vi "OpenScan-packed DRAM-FPGA.vi"() -> ()   [LabVIEW 2015]
uses:
  <vilib>/eio/EIONode/EIONode.xnode
  <vilib>/rvi/eio/common/nirviEmuTemplateMethod_errors.vi
  OpenScan Labview code_20170126/Global_Sample per Frame.vi
  Grobal Variable_Pixel Clock.vi
panel:
  out "Imaging data unpacked for Kalman":u32
  out "Max DRAM address _indicator":u32
  out "Imaging data averaged":u32
  out "Imaging data DRAM address":u32
  in  "Max DRAM address":u32
  in  "Frame number":i32
  out "Number of frames indicator":i32
  out "Waveform output loop count_indicator":i32
  out "Num of elements_indicator":u32=512000
  out "Waiting?":bool=TRUE
  out "Stopping?":bool=TRUE
  out "Frame address_Global":u32
  out "FPGA stop":bool
  out "FPGA loop count":i32
  out "Frams done_indicator":i32
  out "Num of data":u32
  out "Kalman Imaging data address":u32
  out "Display imaging data address":u32
  out "Galvo signal readed_indicator":u32
  in  "Number of frames":i32
  out "Samples acquired":u32
  out "Samples per frame_Global":u32
  out "Frame waveform output finish?":bool
  out "Frame acquisition finish?":bool
  out "image data address indicator":u32
  out "Data indicator":u32
  out "Address counter":u32
  out "Pixel clock_indicator":bool
  out "Frame address_indicator":u32
  out "Averaged image displayed? _indicator":bool
  out "Scanning?":bool
  out "loop count":i32
  out "Display_frames done":i32
  out "Averaged data address":u32
  out "Frame imaging data averaged?":bool
  out "Averaged image displayed?":bool
  in  "Kalman gain":fxp<+,16,1>=0.1015625
  in  "Filter gain":fxp<+,16,0>=0.8000030517578125
  in  "Ready to Scan":bool
  out "Pixel clock (Indicator)":bool
  out "Image averaging done?":bool
  in  "Samples per frame control":u32=262144
  out "Data":u32
  out "Galvo signal readed":u32
  out "Request address":u32
  out "Line clock":bool
  in  "Pixel clock_pulse width(tick)":i32
  in  "Resolution":i32
  in  "Pixel pulse_initial delay":i32
  in  "Frame retrace time":u32 caption="Frame retrace time (ms)"
  in  "Num of undershoot":i32
  in  "Elements per line":i32
  in  "Num of elements":u32
  in  "Pixel time (tick)":i32
  out "Write DRAM done?":bool
  in  "Total elements":u32
  out "Frame Galvo signal write done?":bool
  in  "max addr":u32=1024
  in  "Write DRAM enable?":bool
  in  "Write Frame Galvo signal?":bool
  # "Waveform Data Loading"
  # "Photon Counting"
  # "Waveform Generation"
  # "Controller"
  # "Indicator"
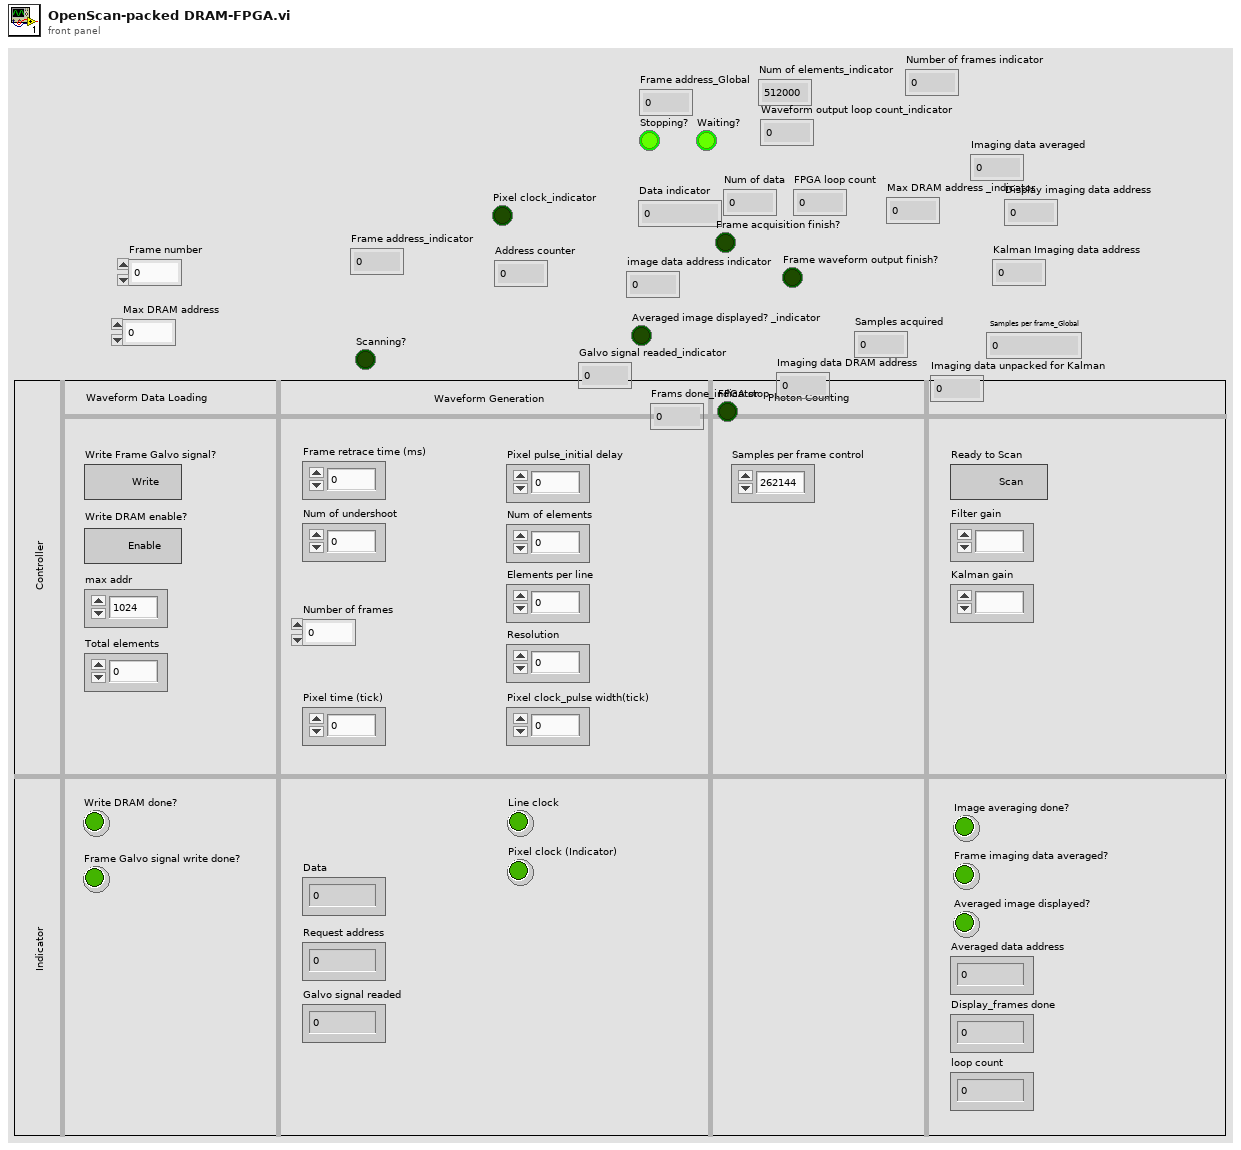
[diagram p1: front panel]
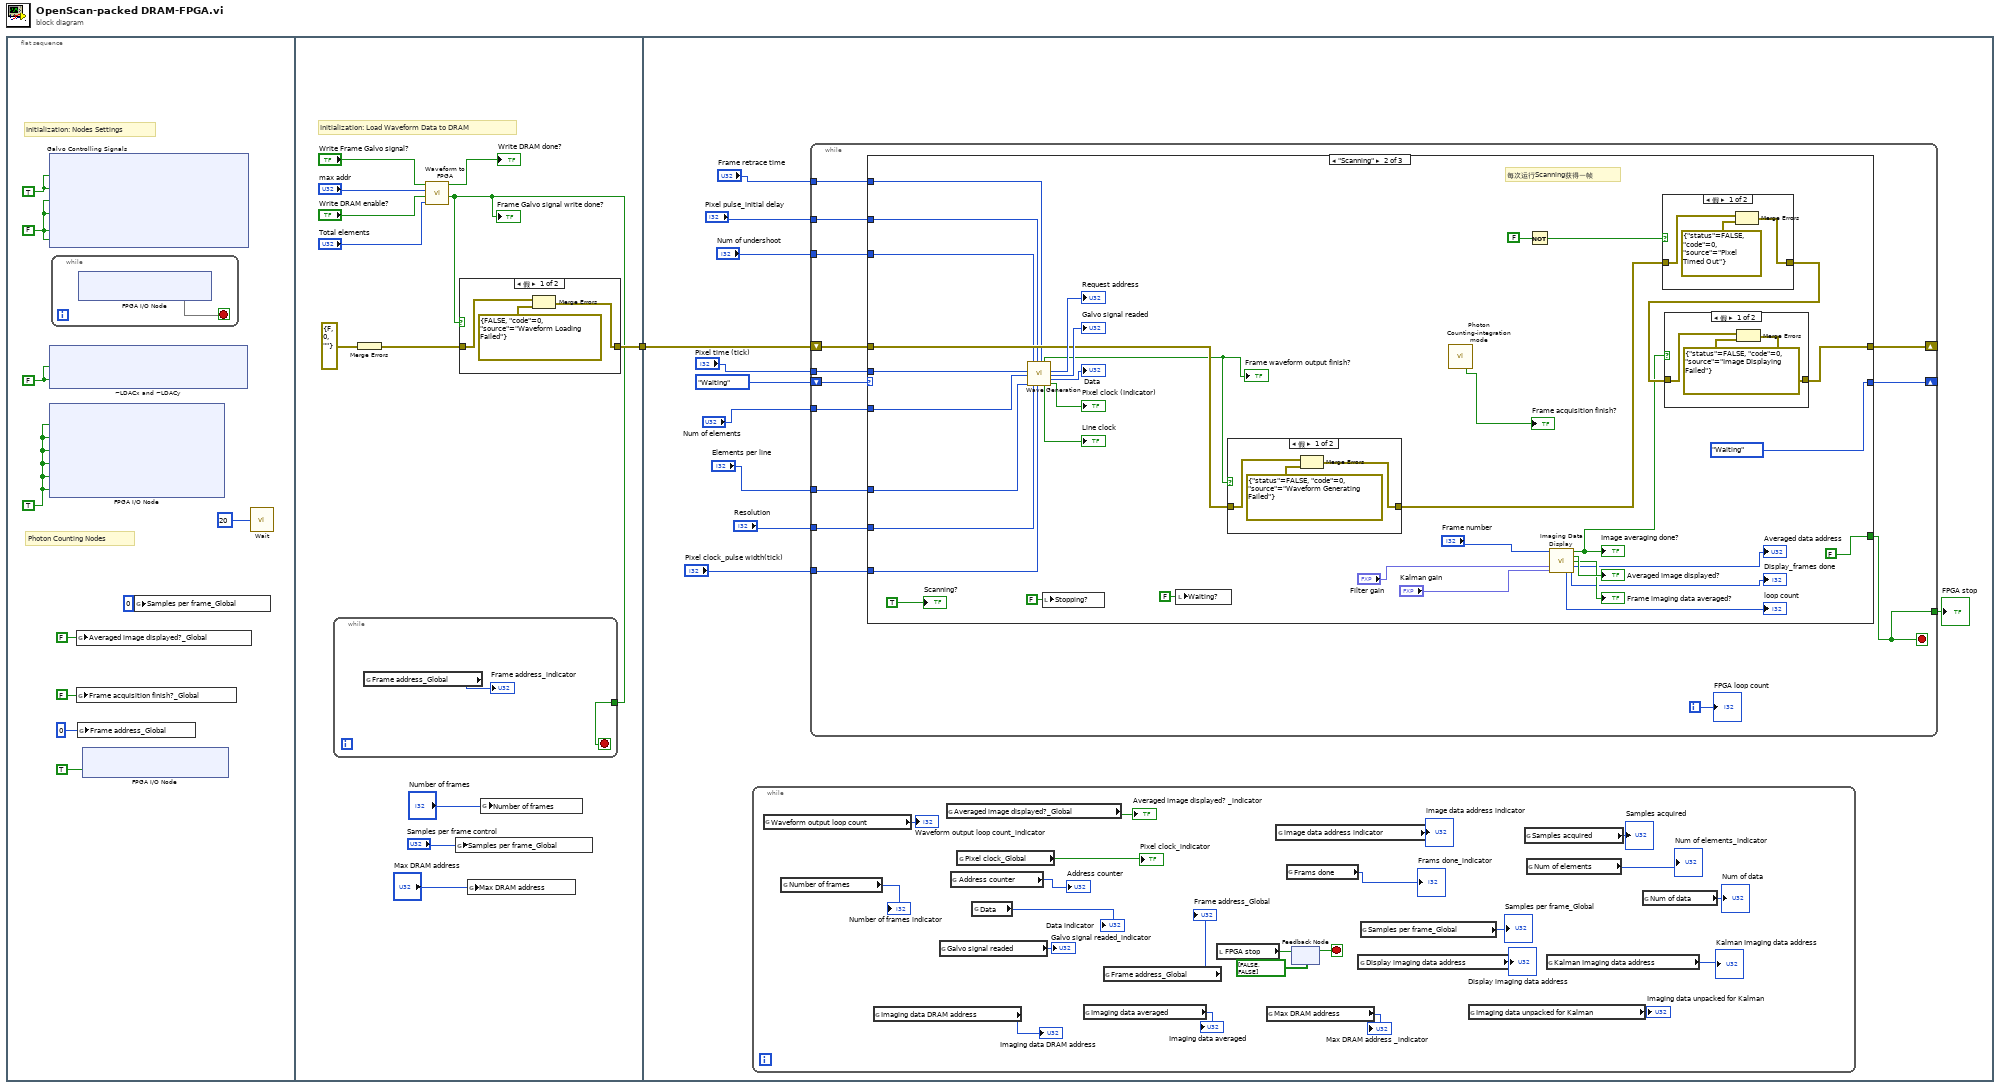
[diagram p0: block diagram]
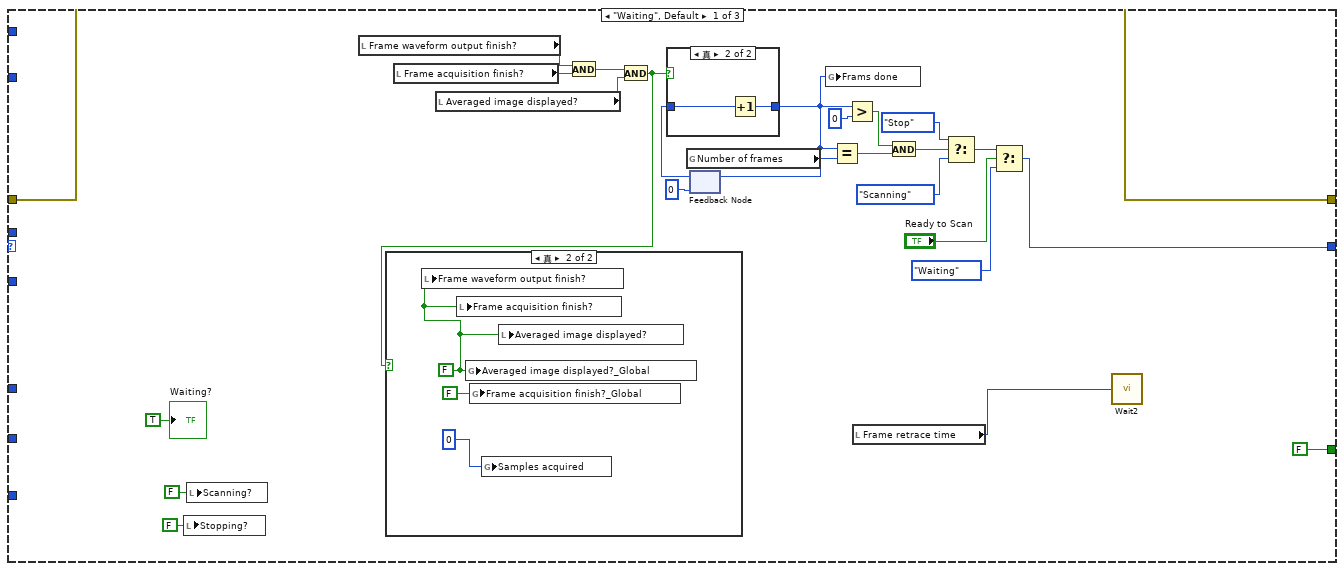
[diagram p3: hidden frame]
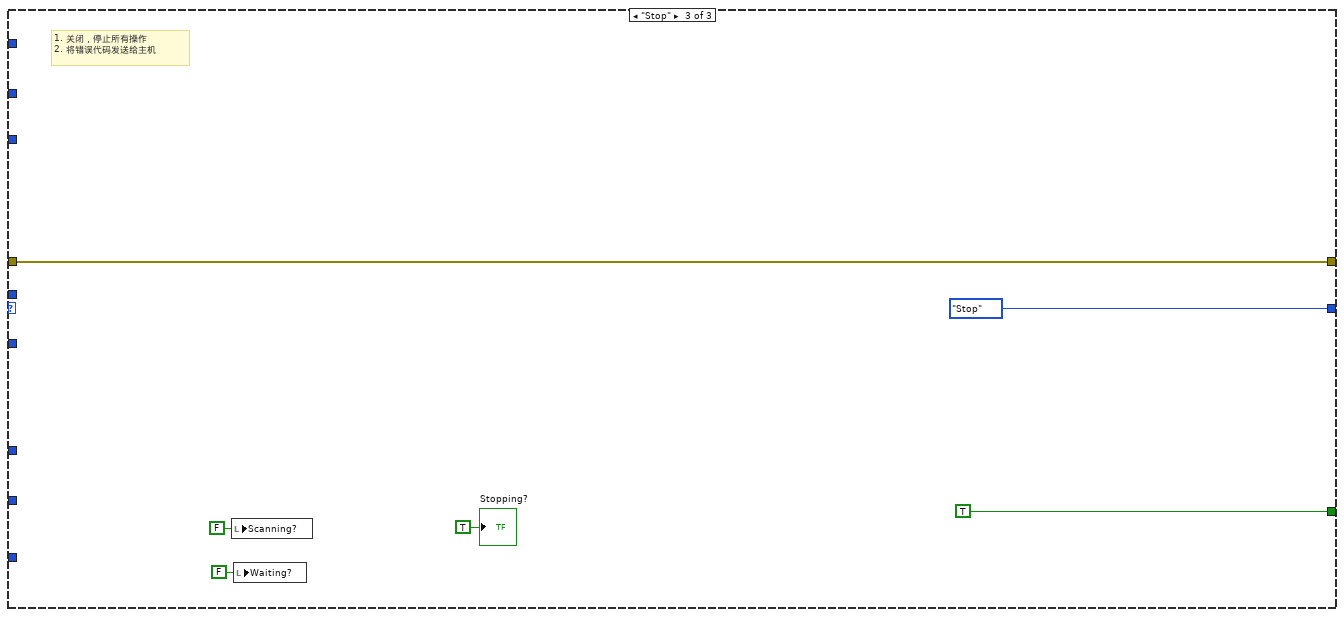
[diagram p9: hidden frame]
diagram:
  n1 = flat-sequence {
    tunnel: [w17] -> w1
    tunnel: w1 -> [w40]
    frame #0 {
      w8 = TRUE ("IO Module\\DDCA_DIO8-15_WE")
      w9 = FALSE ("_LDACx")
      w10 = FALSE ("_CSx")
      w11 = TRUE ("_CLRx")
      # "Photon Counting Nodes"
      # "Initialization: Nodes Settings"
      n2 = xnode "Galvo Controlling Signals"("IO Module\\CLRx(DDCB_DIO0_WRITE)"=w11, "IO Module\\CLRy(DDCB_DIO1_WRITE)"=w11, "IO Module\\CSx(DDCB_DIO2_WRITE)"=w10, "IO Module\\CSy(DDCB_DIO3_WRITE)"=w10, "IO Module\\R_Wx(DDCB_DIO4_WRITE)"=w10, "IO Module\\R_Wy(DDCB_DIO5_WRITE)"=w10) -> ()  [unwired: 6 in, 6 out]
      n3 = xnode "~LDACx and ~LDACy"("IO Module\\LDAx(DDCB_DIO6_WRITE)"=w9, "IO Module\\LDAy(DDCB_DIO7_WRITE)"=w9) -> ()  [unwired: 2 in, 2 out]
      n4 = xnode "FPGA I/O Node"("IO Module\\DDCA_DIO8-15_WE"=w8, "IO Module\\DDCA_DIO16-23_WE"=w8, "IO Module\\DDCB_DIO8-15_WE"=w8, "IO Module\\DDCB_DIO16-23_WE"=w8, "IO Module\\DDCB_DIO0-7_WE"=w8, "IO Module\\DDCB_PFI_WE"=w8) -> ()  [unwired: 6 in, 6 out]
      n5 = while {
        stop <- w12 stop-if-true
        n6 = xnode "FPGA I/O Node"() -> ("IO Module IO Enabled"=w12)  [unwired: 1 in, 1 out]
      }
      n7 = global write "Global_Sample per Frame.vi" "Averaged image displayed?_Global"(FALSE ("Averaged image displayed?")) -> ()
      n8 = global write "Global_Sample per Frame.vi" "Frame acquisition finish?_Global"(FALSE ("Frame acquisition finish?")) -> ()
      n9 = global write "Global_Sample per Frame.vi" "Frame address_Global"(u32 0 ("Frame address")) -> ()
      n10 = xnode "FPGA I/O Node"("IO Module\\DDCA_PFI_WE"=TRUE ("IO Module\\DDCA_DIO8-15_WE")) -> ()  [unwired: 1 in, 1 out]
      n11 = global write "Global_Sample per Frame.vi" "Samples per frame_Global"(u32 0 ("Samples per frame_Global")) -> ()
      n12 = call "Wait"("Count(mSec)"=u32 20) -> ()  [unwired: 1 out]
    }
    frame #1 {
      # "Initialization: Load Waveform Data to DRAM"
      n13 = Merge Errors(errorcluster {"status"=FALSE, "code"=0, "source"=""} ("错误输入")) -> (w18:errorcluster)
      n14 = call "Waveform to FPGA.vi"("Write Frame Galvo signal?"="Write Frame Galvo signal?", "max addr"="max addr", "Write DRAM enable?"="Write DRAM enable?", "Total elements"="Total elements") -> ("Write DRAM done?"=→"Write DRAM done?":bool, "Frame Galvo signal write done?"=w16:bool)  [unwired: 5 in]
      "Frame Galvo signal write done?" <- w16
      n15 = while {
        tunnel: w16 -> [w25]
        stop <- w25 stop-if-true
        n16 = global read "Global_Sample per Frame.vi" "Frame address_Global"() -> (→"Frame address_indicator":u32)
      }
      n17 = global write "Global_Sample per Frame.vi" "Samples per frame_Global"("Samples per frame control") -> ()
      n18 = case shown="假" w16 {
        tunnel: w18 -> [w29 w30]
        tunnel: [w27 w30] -> w17
        frame False {
          n19 = Merge Errors(w29, cluster{bool, "code":i32, "source":string} {FALSE, "code"=0, "source"="Waveform Loading Failed"} ("错误输入")) -> (w27:errorcluster)
        }
        frame True {
        }
      }
      n20 = global write "Global_Sample per Frame.vi" "Max DRAM address"("Max DRAM address") -> ()
      n21 = global write "Global_Sample per Frame.vi" "Number of frames"("Number of frames") -> ()
    }
    frame #2 {
      n22 = while {
        stop <- w50 stop-if-true
        n23 = global read "Global_Sample per Frame.vi" "Waveform output loop count"() -> (→"Waveform output loop count_indicator":i32)
        n24 = global read "Global_Sample per Frame.vi" "Number of frames"() -> (→"Number of frames indicator":i32)
        n25 = global read "Global_Sample per Frame.vi" "Imaging data DRAM address"() -> (→"Imaging data DRAM address":u32)
        n26 = global read "Global_Sample per Frame.vi" "Galvo signal readed"() -> (→"Galvo signal readed_indicator":u32)
        n27 = global read "Global_Sample per Frame.vi" "Averaged image displayed?_Global"() -> (→"Averaged image displayed? _indicator":bool)
        n28 = global read "Global_Sample per Frame.vi" "Address counter"() -> (→"Address counter":u32)
        n29 = global read "Grobal Variable_Pixel Clock.vi" "Pixel clock_Global"() -> (→"Pixel clock_indicator":bool)
        n30 = global read "Global_Sample per Frame.vi" "Data"() -> (→"Data indicator":u32)
        n31 = global read "Global_Sample per Frame.vi" "Imaging data averaged"() -> (→"Imaging data averaged":u32)
        n32 = global read "Global_Sample per Frame.vi" "Frame address_Global"() -> (→"Frame address_Global":u32)
        n33 = local read "FPGA stop"() -> (w53:bool)
        n34 = global read "Global_Sample per Frame.vi" "Max DRAM address"() -> (→"Max DRAM address _indicator":u32)
        n35 = global read "Global_Sample per Frame.vi" "image data address indicator"() -> (→"image data address indicator":u32)
        n36 = global read "Global_Sample per Frame.vi" "Frams done"() -> (→"Frams done_indicator":i32)
        n37 = feedback-in #1(w53) -> ()
        n38 = feedback #1(bool[] [FALSE, FALSE]) -> (w50:bool)
        n39 = global read "Global_Sample per Frame.vi" "Display imaging data address"() -> (→"Display imaging data address":u32)
        n40 = global read "Global_Sample per Frame.vi" "Samples per frame_Global"() -> (→"Samples per frame_Global":u32)
        n41 = global read "Global_Sample per Frame.vi" "Imaging data unpacked for Kalman"() -> (→"Imaging data unpacked for Kalman":u32)
        n42 = global read "Global_Sample per Frame.vi" "Samples acquired"() -> (→"Samples acquired":u32)
        n43 = global read "Global_Sample per Frame.vi" "Num of elements"() -> (→"Num of elements_indicator":u32)
        n44 = global read "Global_Sample per Frame.vi" "Kalman Imaging data address"() -> (→"Kalman Imaging data address":u32)
        n45 = global read "Global_Sample per Frame.vi" "Num of data"() -> (→"Num of data":u32)
      }
      n46 = while {
        shift-right: [w77] -> _
        shift-left: enum16{"Waiting", "Scanning", "Stop"}."Waiting" -> [w78]
        shift-right: [w75] -> _
        shift-left: w40 -> [w76]
        tunnel: "Frame retrace time" -> [w74]
        tunnel: "Pixel pulse_initial delay" -> [w73]
        tunnel: "Num of undershoot" -> [w72]
        tunnel: "Pixel time (tick)" -> [w71]
        tunnel: "Num of elements" -> [w70]
        tunnel: "Elements per line" -> [w69]
        tunnel: "Resolution" -> [w68]
        tunnel: "Pixel clock_pulse width(tick)" -> [w67]
        tunnel: [w65] -> w31
        i -> [w66]
        stop <- w65 stop-if-true
        n47 = case shown="\"Scanning\"" w78 {
          tunnel: [w102 enum16{"Waiting", "Scanning", "Stop"}."Waiting" enum16{"Waiting", "Scanning", "Stop"}."Stop"] -> w77
          tunnel: w76 -> [w103 w139 w162]
          tunnel: [w103 w133 w162] -> w75
          tunnel: w74 -> [_ w126 _]
          tunnel: w73 -> [_ w125 _]
          tunnel: w72 -> [_ w124 _]
          tunnel: w71 -> [_ w123 _]
          tunnel: w70 -> [_ w122 _]
          tunnel: w69 -> [_ w121 _]
          tunnel: w68 -> [_ w120 _]
          tunnel: w67 -> [_ w119 _]
          tunnel: [FALSE FALSE TRUE] -> w65
          frame "Waiting", Default {
            n48 = local write "Stopping?"(FALSE ("Stopping?")) -> ()
            n49 = local write "Scanning?"(FALSE ("Scanning?")) -> ()
            n50 = local read "Frame waveform output finish?"() -> (w94:bool)
            n51 = local read "Frame acquisition finish?"() -> (w95:bool)
            n52 = local read "Averaged image displayed?"() -> (w96:bool)
            n53 = And(x=w94, y=w95) -> (x .and. y?=w97:bool)
            n54 = And(x=w97, y=w96) -> (x .and. y?=w82:bool)
            n55 = case shown="真" w82 {
              frame False {
              }
              frame True {
                w104 = FALSE ("Averaged image displayed?")
                n56 = local write "Frame waveform output finish?"(w104) -> ()
                n57 = local write "Frame acquisition finish?"(w104) -> ()
                n58 = global write "Global_Sample per Frame.vi" "Averaged image displayed?_Global"(w104) -> ()
                n59 = global write "Global_Sample per Frame.vi" "Frame acquisition finish?_Global"(FALSE ("Frame acquisition finish?")) -> ()
                n60 = global write "Global_Sample per Frame.vi" "Samples acquired"(u32 0 ("Frame address")) -> ()
                n61 = local write "Averaged image displayed?"(w104) -> ()
              }
            }
            n62 = global read "Global_Sample per Frame.vi" "Number of frames"() -> (w89:i32)
            n63 = feedback #2(0) -> (w98:i32)
            n64 = case shown="真" w82 {
              tunnel: w98 -> [w107 w108]
              tunnel: [w107 w109] -> w88
              frame False {
              }
              frame True {
                n65 = Increment(x=w108) -> (x+1=w109:i32)
              }
            }
            n66 = feedback-in #2(w88) -> ()
            n67 = global write "Global_Sample per Frame.vi" "Frams done"(w88) -> ()
            n68 = Equal?(x=w88, y=w89) -> (x = y?=w85:bool)
            n69 = Greater?(x=w88, y=0) -> (0:w86:bool)
            n70 = local read "Frame retrace time"() -> (w83:u32)
            n71 = And(x=w86, y=w85) -> (x .and. y?=w84:bool)
            n72 = Select(t=enum16{"Waiting", "Scanning", "Stop"}."Stop", s=w84, f=enum16{"Waiting", "Scanning", "Stop"}."Scanning") -> (s? t:f=w90:enum16{"Waiting", "Scanning", "Stop"})
            n73 = Select(t=w90, s="Ready to Scan", f=enum16{"Waiting", "Scanning", "Stop"}."Waiting") -> (s? t:f=w102:enum16{"Waiting", "Scanning", "Stop"})
            n74 = call "Wait2"("Count(mSec)"=w83) -> ()  [unwired: 1 out]
            "Waiting?" <- TRUE
          }
          frame "Scanning" {
            # "每次运行Scanning获得一帧"
            n75 = call "Wave Generation.vi"("Pixel time (tick)"=w123, "Num of elements"=w122, "Elements per line"=w121, "Num of undershoot"=w124, "Resolution"=w120, "Pixel pulse_initial delay"=w125, "Pixel clock_pulse width(tick)"=w119, "Frame retrace time"=w126) -> ("Frame waveform output finish?"=w118:bool, "Line clock"=→"Line clock":bool, "Request address"=→"Request address":u32, "Galvo signal readed"=→"Galvo signal readed":u32, "Data"=→"Data":u32, "Pixel clock"=→"Pixel clock (Indicator)":bool)  [unwired: 6 in]
            "Frame waveform output finish?" <- w118
            n76 = local write "Stopping?"(FALSE ("Stopping?")) -> ()
            n77 = local write "Waiting?"(FALSE ("Waiting?")) -> ()
            n78 = case shown="假" w118 {
              tunnel: w139 -> [w155 w156]
              tunnel: [w153 w156] -> w138
              frame False {
                n79 = Merge Errors(w155, errorcluster {"status"=FALSE, "code"=0, "source"="Waveform Generating Failed"} ("错误输入")) -> (w153:errorcluster)
              }
              frame True {
              }
            }
            n80 = call "Photon Counting-integration mode.vi"() -> ("Frame acquisition finish?"=→"Frame acquisition finish?":bool)  [unwired: 19 in]
            n81 = Not(x=FALSE) -> (.not. x?=w137:bool)
            n82 = call "Imaging Data Display.vi"("Frame number"="Frame number", "Filter gain"="Filter gain", "Kalman gain"="Kalman gain") -> ("Image averaging done?"=w135:bool, "Averaged image displayed?"=→"Averaged image displayed?":bool, "Frame imaging data Averaged?"=→"Frame imaging data averaged?":bool, "Averaged data address"=→"Averaged data address":u32, "loop count"=→"loop count":i32, "Display_frames done"=→"Display_frames done":i32)  [unwired: 7 in]
            "Image averaging done?" <- w135
            n83 = case shown="假" w137 {
              tunnel: w138 -> [w151 w152]
              tunnel: [w149 w152] -> w136
              frame False {
                n84 = Merge Errors(w151, errorcluster {"status"=FALSE, "code"=0, "source"="Pixel Timed Out"} ("错误输入")) -> (w149:errorcluster)
              }
              frame True {
              }
            }
            n85 = case shown="假" w135 {
              tunnel: w136 -> [w147 w148]
              tunnel: [w145 w148] -> w133
              frame False {
                n86 = Merge Errors(w147, errorcluster {"status"=FALSE, "code"=0, "source"="Image Displaying Failed"} ("错误输入")) -> (w145:errorcluster)
              }
              frame True {
              }
            }
            "Scanning?" <- TRUE
          }
          frame "Stop" {
            # "1. 关闭，停止所有操作\n2. 将错误代码发送给主机"
            n87 = local write "Scanning?"(FALSE ("Scanning?")) -> ()
            n88 = local write "Waiting?"(FALSE ("Waiting?")) -> ()
            "Stopping?" <- TRUE
          }
        }
        "FPGA loop count" <- w66
      }
      "FPGA stop" <- w31
    }
  }
